vi "VI Tree.vi"   [LabVIEW 2020, in "Agilent 6XXX Series.lvlib"]
doc: "The VI Tree shows all of the VI's in the driver.\n\nThis is the instrument driver for the HP 6XXXA Series DC Power Supplies\nThe driver supports the following: HP 6030A, 6031A, 6032A, 6033A, 6035A, 6038A, 6621A, 6622A, 6623A, 6624A, 6627A, 6632A, 6633A, and 6634A DC Power Supplies. \nThe Instrument Driver Revision: is \"Rev 1.0.1, 06/97, LV 4.1\", the Instrument Firmware Revision is Not Available"
uses:
  <instrlib>/Agilent 6XXX Series/Agilent 6XXX Series.lvlib
panel:
  # "See Diagram Box\nfor VI Tree"
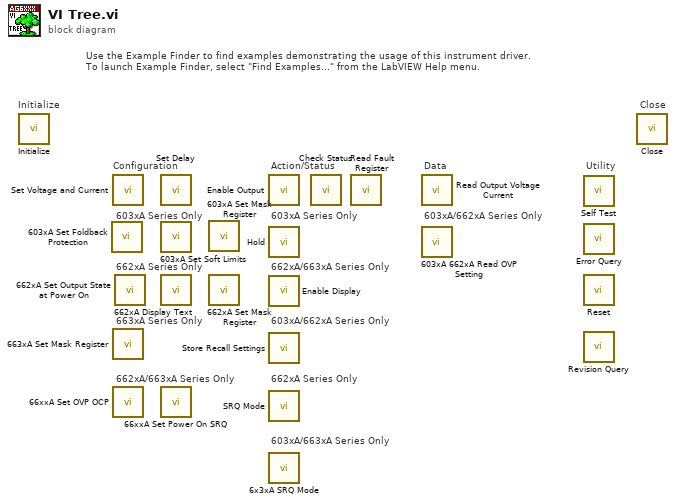
[diagram p0: block diagram]
diagram:
  # "Close"
  # "603xA/662xA Series Only"
  # "662xA Series Only"
  # "662xA/663xA Series Only"
  # "603xA Series Only"
  # "Utility"
  # "603xA/663xA Series Only"
  # "Data"
  # "603xA/662xA Series Only"
  # "Action/Status"
  # "662xA/663xA Series Only"
  # "663xA Series Only"
  # "662xA Series Only"
  # "603xA Series Only"
  # "Configuration"
  # "Initialize"
  # "Use the Example Finder to find examples demonstrating the usage of this instrument driver.\nTo launch Example Finder, select \"Find Examples...\" from the LabVIEW Help menu."
  n1 = call <instrlib>:"Initialize.vi"() -> ()  [unwired: 10 in, 2 out]
  n2 = call <instrlib>:"603xA Set Foldback Protection.vi"() -> ()  [unwired: 10 in, 2 out]
  n3 = call <instrlib>:"Set Voltage and Current.vi"() -> ()  [unwired: 10 in, 2 out]
  n4 = call <instrlib>:"663xA Set Mask Register.vi"() -> ()  [unwired: 18 in, 2 out]
  n5 = call <instrlib>:"66xxA Set OVP OCP.vi"() -> ()  [unwired: 10 in, 2 out]
  n6 = call <instrlib>:"662xA Set Output State at Power On.vi"() -> ()  [unwired: 10 in, 2 out]
  n7 = call <instrlib>:"Set Delay.vi"() -> ()  [unwired: 10 in, 2 out]
  n8 = call <instrlib>:"603xA Set Soft Limits.vi"() -> ()  [unwired: 10 in, 2 out]
  n9 = call <instrlib>:"662xA Display Text.vi"() -> ()  [unwired: 10 in, 2 out]
  n10 = call <instrlib>:"66xxA Set Power On SRQ.vi"() -> ()  [unwired: 10 in, 2 out]
  n11 = call <instrlib>:"603xA Set Mask Register.vi"() -> ()  [unwired: 14 in, 2 out]
  n12 = call <instrlib>:"662xA Set Mask Register.vi"() -> ()  [unwired: 14 in, 2 out]
  n13 = call <instrlib>:"Enable Output.vi"() -> ()  [unwired: 10 in, 2 out]
  n14 = call <instrlib>:"Hold.vi"() -> ()  [unwired: 10 in, 2 out]
  n15 = call <instrlib>:"Enable Display.vi"() -> ()  [unwired: 10 in, 2 out]
  n16 = call <instrlib>:"Store Recall Settings.vi"() -> ()  [unwired: 10 in, 2 out]
  n17 = call <instrlib>:"SRQ Mode.vi"() -> ()  [unwired: 10 in, 2 out]
  n18 = call <instrlib>:"6x3xA SRQ Mode.vi"() -> ()  [unwired: 10 in, 2 out]
  n19 = call <instrlib>:"Check Status.vi"() -> ()  [unwired: 9 in, 3 out]
  n20 = call <instrlib>:"Read Fault Register.vi"() -> ()  [unwired: 9 in, 3 out]
  n21 = call <instrlib>:"Read Output Voltage Current.vi"() -> ()  [unwired: 8 in, 4 out]
  n22 = call <instrlib>:"603xA 662xA Read OVP Setting.vi"() -> ()  [unwired: 9 in, 3 out]
  n23 = call <instrlib>:"Self Test.vi"() -> ()  [unwired: 8 in, 4 out]
  n24 = call <instrlib>:"Error Query.vi"() -> ()  [unwired: 8 in, 4 out]
  n25 = call <instrlib>:"Reset.vi"() -> ()  [unwired: 10 in, 2 out]
  n26 = call <instrlib>:"Revision Query.vi"() -> ()  [unwired: 8 in, 4 out]
  n27 = call <instrlib>:"Close.vi"() -> ()  [unwired: 11 in, 1 out]
